vi "每列有效平均值.vi"(10 "测试数组":string[][](array[string])) -> (2 "平均混响时间":dbl[](array[numeric]) format="%#.2g", 3 "混响2D数值":dbl[][](array[numeric]))   [LabVIEW 2020]
panel:
  out "每列有效数量":i32[](array[numeric])
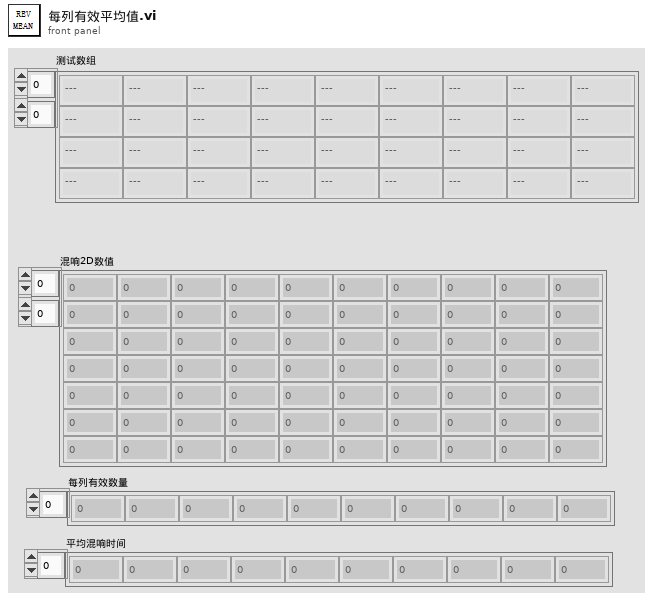
[diagram p1: front panel]
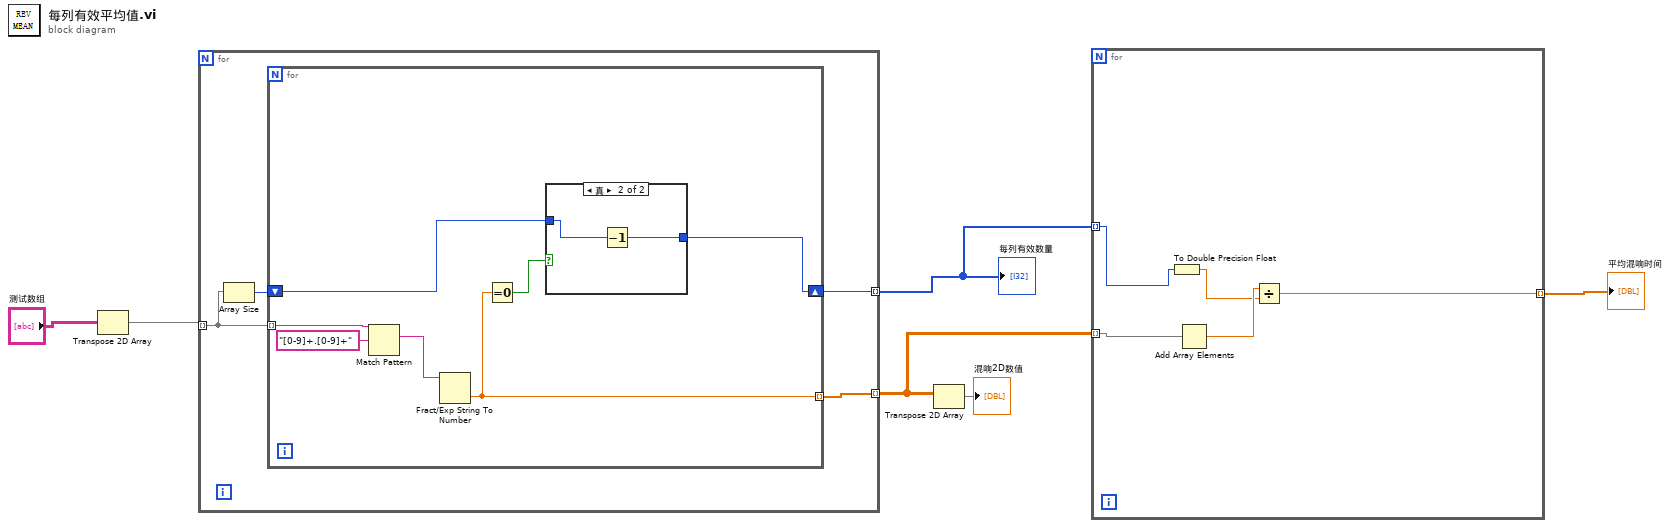
[diagram p0: block diagram]
diagram:
  n1 = Transpose 2D Array(2D array="测试数组") -> (transposed array=w5:string[][])
  n2 = for {
    tunnel: w5 -> [w9] mode=indexing
    tunnel: [w10] -> w3 mode=indexing
    tunnel: [w7] -> w2 mode=indexing
    n3 = Array Size(array=w9) -> (size(s)=w8:i32)
    n4 = for {
      tunnel: [w14] -> w10 mode=indexing
      tunnel: w9 -> [w16] mode=indexing
      shift-right: [w11] -> w7
      shift-left: w8 -> [w12]
      n5 = Match Pattern(string=w16, regular expression="[0-9]+.[0-9]+" ("正则表达式")) -> (match substring=w15:string)  [unwired: 1 in, 3 out]
      n6 = Fract/Exp String To Number(string=w15) -> (number=w14:dbl)  [unwired: 3 in, 1 out]
      n7 = Equal To 0?(x=w14) -> (x = 0?=w13:bool)
      n8 = case shown="真" w13 {
        tunnel: w12 -> [w18 w20]
        tunnel: [w18 w19] -> w11
        frame False {
        }
        frame True {
          n9 = Decrement(x=w20) -> (x-1=w19:i32)
        }
      }
    }
  }
  "每列有效数量" <- w2
  n10 = Transpose 2D Array(2D array=w3) -> (transposed array=→"混响2D数值":dbl[][])
  n11 = for {
    tunnel: w3 -> [w25] mode=indexing
    tunnel: w2 -> [w22] mode=indexing
    tunnel: [w23] -> w1 mode=indexing
    n12 = To Double Precision Float(number=w22) -> (double precision float=w21:dbl)
    n13 = Add Array Elements(numeric array=w25) -> (sum=w24:dbl)
    n14 = Divide(x=w24, y=w21) -> (x/y=w23:dbl)
  }
  "平均混响时间" <- w1
